vi "DAQ AI trig buff ch 4 5.vi"(0 "device name":tag="Dev1", 1 "timeout (s)":dbl=1.0 format="%0.2f", 2 "stop (T)":bool=TRUE, 5 "number of samples (1000)":i32=1000, 9 "rate (100K)":dbl=100000.0, 11 "error in":errorcluster, 12 "physical channel":string[](array[string])=["ai4", "ai5"], 13 "channel name":string[](array[string])=["drive signal", "RC response"]) -> (4 "device name out":tag="Dev1", 8 "data waveforms":waveform(dbl)[](array[waveform]), 15 "error out":errorcluster)   [LabVIEW 2019]
doc: "DAQmx NI ELVIS \nSynchronous bufffered AI\ntriggered\nchannels 4 5\nbug drive and RC response\n\ncreated with DAQmx assistant\n\nPaul K Dixon\nP3600\nCSUSB Physics\n\nCreates, edits, and runs tasks using NI-DAQmx. Refer to the NI-DAQmx Readme for a complete listing of devices NI-DAQmx supports.\n\nWhen you place this Express VI on the block diagram, the DAQ Assistant launches to create a new task. After you create a task, you can double-click the DAQ Assistant Express VI to edit that task. For continuous measurement or generation, place a while loop around the DAQ Assistant Express VI."
uses:
  <vilib>/DAQmx/read.llb/DAQmx Read.vi
  <vilib>/DAQmx/read.llb/DAQmx Read (Analog 1D Wfm NChan NSamp).vi
  <vilib>/DAQmx/create/channels.llb/DAQmx Create Channel (TEDS-AI-Voltage-Basic).vi
  <vilib>/DAQmx/create/channels.llb/DAQmx Create Channel (AI-Voltage-Basic).vi
  <vilib>/DAQmx/configure/timing.llb/DAQmx Timing (Sample Clock).vi
  <vilib>/DAQmx/configure/trigger.llb/DAQmx Trigger.vi
  <vilib>/DAQmx/configure/trigger.llb/DAQmx Start Trigger (Analog Edge).vi
  <vilib>/DAQmx/miscellaneous.llb/DAQmx Fill In Error Info.vi
panel:
  in  "source":string="drive signal"
  in  "slope":i32(ring)=10171 items=["Rising"=10280, "Falling"=10171]
  in  "level":dbl=2.0 format="%0.2f"
  out "data":dynamicdata(graph)
  # "Trigger Settings"
  # "DAQmx NI ELVIS \nSynchronous bufffered AI\ntriggered\nchannels 4 5\nbug drive and RC response"
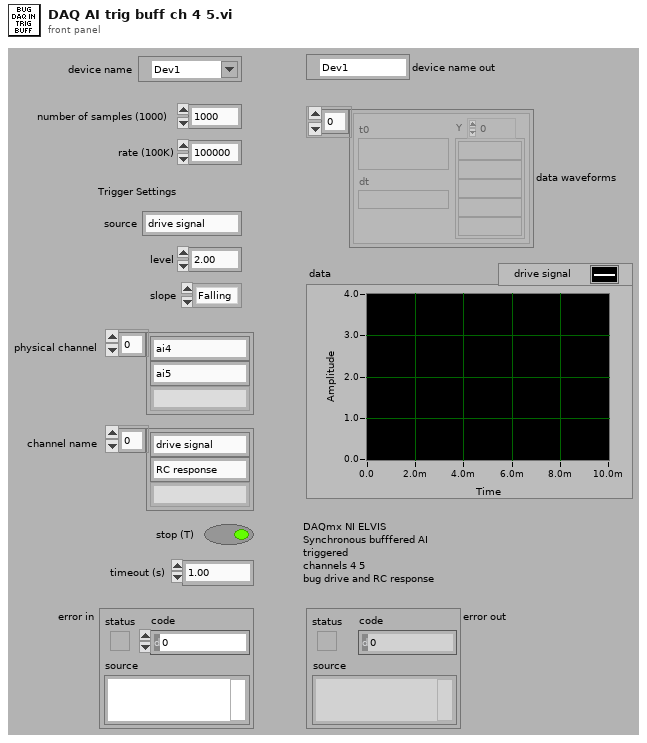
[diagram p1: front panel]
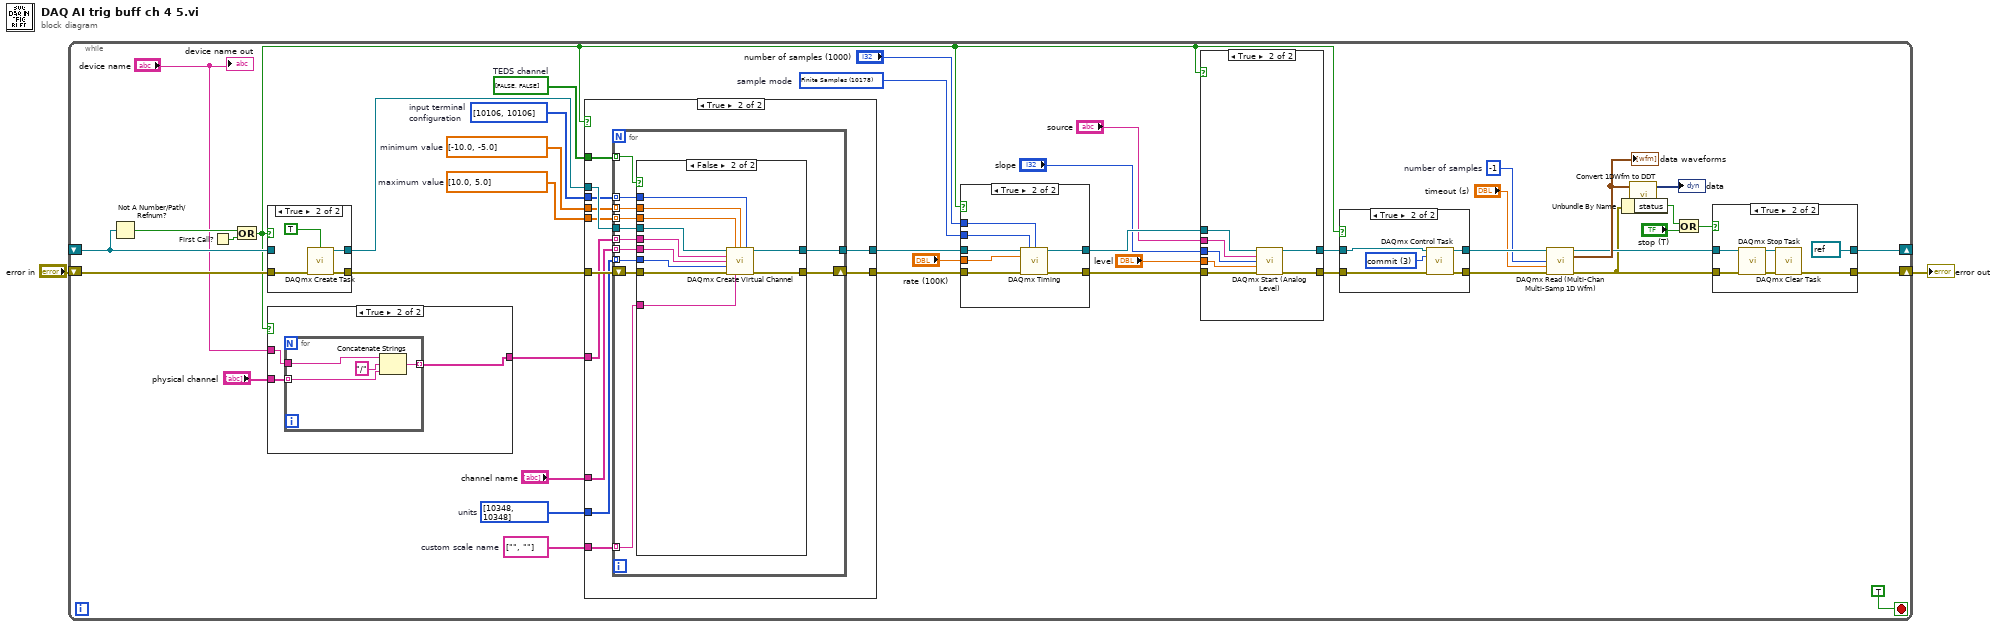
[diagram p0: block diagram]
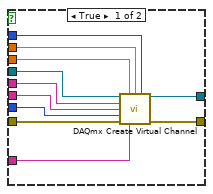
[diagram p7: hidden frame]
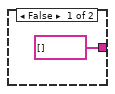
[diagram p8: hidden frame]
diagram:
  n1 = while {
    shift-right: [w9] -> _
    shift-left: _ -> [w42]
    shift-right: [w7] -> w1
    shift-left: "error in" -> [w43]
    stop <- TRUE stop-if-true
    w13 = -1  # number of samples
    w24 = 10178 items=["Finite Samples"=10178, "Continuous Samples"=10123, "Hardware Timed Single Point"=12522]  # sample mode
    w29 = bool[] [FALSE, FALSE]  # TEDS channel
    w30 = string[] ["", ""]  # custom scale name
    w31 = i32[] [10348, 10348] items=["Volts"=10348, "From TEDS"=12516, "From Custom Scale"=10065]  # units
    w34 = dbl[] [10.0, 5.0]  # maximum value
    w35 = dbl[] [-10.0, -5.0]  # minimum value
    w36 = i32[] [10106, 10106] items=["default"=-1, "RSE"=10083, "NRSE"=10078, "Differential"=10106, "Pseudodifferential"=12529]  # input terminal configuration
    n2 = Not A Number/Path/Refnum?(number/path/refnum=w42) -> (NaN/Path/Refnum?=w41:bool)
    n3 = First Call?() -> (First Call?: T/F=w44:bool)
    n4 = Or(x=w41, y=w44) -> (x .or. y?=w18:bool)
    n5 = case shown="True" w18 {
      tunnel: [w136 w140] -> w38
      tunnel: w42 -> [w136 _]
      tunnel: [w135 w139] -> w37
      tunnel: w43 -> [w135 w137]
      frame False {
      }
      frame True {
        n6 = call <vilib>:"DAQmx Create Task.vi"("auto cleanup"=TRUE, "error in"=w137) -> ("task out"=w140:refnum<k21>, "error out"=w139:errorcluster)  [unwired: 12 in]
      }
    }
    n7 = case shown="True" w18 {
      tunnel: [string[] [] w130] -> w33
      tunnel: "device name" -> [_ w129]
      tunnel: "physical channel" -> [_ w128]
      frame False {
      }
      frame True {
        n8 = for {
          tunnel: [w134] -> w130 mode=indexing
          tunnel: w129 -> [w133]
          tunnel: w128 -> [w131] mode=indexing
          n9 = Concatenate Strings(w133, "/" ("string"), w131) -> (w134:string)
        }
      }
    }
    n10 = case shown="True" w18 {
      tunnel: [w80 w90] -> w28
      tunnel: w38 -> [w80 w92]
      tunnel: [w79 w89] -> w27
      tunnel: w37 -> [w79 w91]
      tunnel: w36 -> [_ w88]
      tunnel: w35 -> [_ w87]
      tunnel: w34 -> [_ w86]
      tunnel: w33 -> [_ w85]
      tunnel: "channel name" -> [_ w84]
      tunnel: w31 -> [_ w83]
      tunnel: w30 -> [_ w82]
      tunnel: w29 -> [_ w81]
      frame False {
      }
      frame True {
        n11 = for {
          tunnel: w92 -> [w104]
          tunnel: [w102] -> w90
          tunnel: w88 -> [w100] mode=indexing
          tunnel: w87 -> [w99] mode=indexing
          tunnel: w86 -> [w98] mode=indexing
          tunnel: w85 -> [w97] mode=indexing
          tunnel: w84 -> [w96] mode=indexing
          tunnel: w83 -> [w95] mode=indexing
          tunnel: w82 -> [w94] mode=indexing
          shift-right: [w101] -> w89
          shift-left: w91 -> [w103]
          tunnel: w81 -> [w93] mode=indexing
          n12 = case shown="False" w93 {
            tunnel: w104 -> [w115 w126]
            tunnel: w103 -> [w114 w125]
            tunnel: [w113 w124] -> w102
            tunnel: [w112 w123] -> w101
            tunnel: w100 -> [w111 w122]
            tunnel: w99 -> [w110 w121]
            tunnel: w98 -> [w109 w120]
            tunnel: w97 -> [w108 w119]
            tunnel: w96 -> [w107 w118]
            tunnel: w95 -> [w106 w117]
            tunnel: w94 -> [w105 w116]
            frame True {
              n13 = call-poly <vilib>:"DAQmx Create Virtual Channel.vi"("task in"=w115, "maximum value"=w109, "minimum value"=w110, "input terminal configuration"=w111, "physical channels"=w108, "name to assign"=w107, "units"=w106, "error in"=w114, "custom scale name"=w105) -> ("task out"=w113:refnum<k21>, "error out"=w112:errorcluster)  [unwired: 5 in]
            }
            frame False {
              n14 = call-poly <vilib>:"DAQmx Create Virtual Channel.vi"("task in"=w126, "maximum value"=w120, "minimum value"=w121, "input terminal configuration"=w122, "physical channels"=w119, "name to assign"=w118, "units"=w117, "error in"=w125, "custom scale name"=w116) -> ("task out"=w124:refnum<k21>, "error out"=w123:errorcluster)  [unwired: 5 in]
            }
          }
        }
      }
    }
    n15 = case shown="True" w18 {
      tunnel: [w71 w73] -> w23
      tunnel: w28 -> [w71 w76]
      tunnel: [w70 w72] -> w22
      tunnel: w27 -> [w70 w74]
      tunnel: "number of samples (1000)" -> [_ w78]
      tunnel: w24 -> [_ w77]
      tunnel: "rate (100K)" -> [_ w75]
      frame False {
      }
      frame True {
        n16 = call-poly <vilib>:"DAQmx Timing.vi"("task/channels in"=w76, "sample mode"=w77, "samples per channel"=w78, "rate"=w75, "error in"=w74) -> ("task out"=w73:refnum<k21>, "error out"=w72:errorcluster)  [unwired: 9 in]
      }
    }
    n17 = case shown="True" w18 {
      tunnel: [w62 w67] -> w17
      tunnel: w23 -> [w62 w69]
      tunnel: [w61 w66] -> w16
      tunnel: w22 -> [w61 w68]
      tunnel: "source" -> [_ w65]
      tunnel: "slope" -> [_ w64]
      tunnel: "level" -> [_ w63]
      frame False {
      }
      frame True {
        n18 = call-poly "DAQmx Start (Analog Level).vi"("task/channels in"=w69, "source"=w65, "slope"=w64, "level"=w63, "error in"=w68) -> ("task out"=w67:refnum<k21>, "error out"=w66:errorcluster)  [unwired: 9 in]
      }
    }
    n19 = case shown="True" w18 {
      tunnel: [w55 w59] -> w15
      tunnel: w17 -> [w55 w60]
      tunnel: [w54 w57] -> w14
      tunnel: w16 -> [w54 w58]
      frame False {
      }
      frame True {
        w56 = 3 items=["verify"=2, "reserve"=4, "commit"=3, "unreserve"=5, "abort"=6] ("action")
        n20 = call <vilib>:"DAQmx Control Task.vi"("task/channels in"=w60, "action"=w56, "error in"=w58) -> ("task out"=w59:refnum<k21>, "error out"=w57:errorcluster)  [unwired: 11 in]
      }
    }
    n21 = call-poly "DAQmx Read (Multi-Chan Multi-Samp 1D Wfm).vi"("task/channels in"=w15, "number of samples per channel"=w13, "timeout"="timeout (s)", "error in"=w14) -> ("task out"=w8:refnum<k21>, "data"=w12:waveform(dbl)[], "error out"=w6:errorcluster)  [unwired: 9 in]
    "data waveforms" <- w12
    n22 = Unbundle By Name(w6) -> ("status"=w5:bool)
    n23 = call <vilib>:"Convert 1DWfm to DDT.vi"("Array of Waveforms"=w12) -> ("Dynamic Data Type"=→"data":dynamicdata)  [unwired: 3 in]
    n24 = Or(x=w5, y="stop (T)") -> (x .or. y?=w3:bool)
    n25 = case shown="True" w3 {
      tunnel: [w47 refnum<k21> refnum ("task in")] -> w9
      tunnel: w8 -> [w47 w53]
      tunnel: [w46 w50] -> w7
      tunnel: w6 -> [w46 w52]
      frame False {
      }
      frame True {
        n26 = call <vilib>:"DAQmx Stop Task.vi"("task/channels in"=w53, "error in"=w52) -> ("task out"=w49:refnum<k21>, "error out"=w51:errorcluster)  [unwired: 12 in]
        n27 = call <vilib>:"DAQmx Clear Task.vi"("task in"=w49, "error in"=w51) -> ("error out"=w50:errorcluster)  [unwired: 13 in]
      }
    }
    "device name out" <- "device name"
  }
  "error out" <- w1
